vi "q1.vi"() -> ()   [LabVIEW 2015]
panel:
  out "Sin wave":dbl[](graph)=[0.0, 0.06279051952931337, 0.12533323356430426, 0.1873813145857246, 0.2486898871648548, 0.3090169943749474, 0.3681245526846779, 0.4257792915650727, 0.4817536741017153, 0.5358267949789967, 0.5877852522924731, 0.6374239897486896, 0.6845471059286886, 0.7289686274214116, 0.7705132427757893, 0.8090169943749475, 0.8443279255020151, 0.8763066800438637, 0.9048270524660196, 0.9297764858882513, 0.9510565162951535, 0.9685831611286311, 0.9822872507286886, 0.9921147013144779, 0.9980267284282716, 1.0, 0.9980267284282716, 0.9921147013144778, 0.9822872507286886, 0.9685831611286312, 0.9510565162951536, 0.9297764858882515, 0.9048270524660195, 0.8763066800438635, 0.844327925502015, 0.8090169943749475, 0.7705132427757893, 0.7289686274214114, 0.6845471059286888, 0.6374239897486899, 0.5877852522924732, 0.5358267949789967, 0.4817536741017156, 0.4257792915650729, 0.36812455268467814, 0.3090169943749475, 0.24868988716485482, 0.18738131458572457, 0.12533323356430454, 0.06279051952931358, 1.2246467991473532e-16, -0.06279051952931335, -0.12533323356430429, -0.18738131458572477, -0.24868988716485502, -0.30901699437494773, -0.3681245526846783, -0.42577929156507266, -0.481753674101715, -0.5358267949789964, -0.587785252292473, -0.6374239897486896, -0.6845471059286887, -0.7289686274214113, -0.7705132427757894, -0.8090169943749473, -0.8443279255020153, -0.8763066800438636, -0.9048270524660198, -0.9297764858882515, -0.9510565162951535, -0.968583161128631, -0.9822872507286887, -0.9921147013144778, -0.9980267284282716, -1.0, -0.9980267284282716, -0.9921147013144779, -0.9822872507286887, -0.9685831611286311, -0.9510565162951536, -0.9297764858882512, -0.9048270524660196, -0.8763066800438634, -0.8443279255020155, -0.8090169943749476, -0.7705132427757896, -0.7289686274214116, -0.684547105928689, -0.6374239897486896, -0.5877852522924734, -0.5358267949789963, -0.4817536741017153, -0.4257792915650722, -0.36812455268467786, -0.3090169943749477, -0.24868988716485535, -0.18738131458572468, -0.12533323356430465, -0.06279051952931326, -2.4492935982947064e-16, 0.06279051952931278, 0.12533323356430418, 0.1873813145857242, 0.24868988716485488, 0.3090169943749472, 0.3681245526846782, 0.42577929156507255, 0.48175367410171566, 0.5358267949789967, 0.5877852522924736, 0.63742398974869, 0.6845471059286892, 0.7289686274214119, 0.7705132427757893, 0.8090169943749478, 0.8443279255020147, 0.8763066800438631, 0.9048270524660194, 0.9297764858882511, 0.9510565162951535, 0.968583161128631, 0.9822872507286886, 0.9921147013144778, 0.9980267284282716, 1.0, 0.9980267284282716, 0.9921147013144779, 0.9822872507286886, 0.9685831611286311, 0.9510565162951536, 0.9297764858882517, 0.9048270524660192, 0.8763066800438634, 0.8443279255020151, 0.8090169943749476, 0.7705132427757886, 0.728968627421411, 0.6845471059286884, 0.6374239897486897, 0.5877852522924734, 0.5358267949789972, 0.4817536741017162, 0.42577929156507394, 0.368124552684678, 0.3090169943749478, 0.2486898871648555, 0.18738131458572568, 0.1253332335643039, 0.06279051952931339, 3.6739403974420594e-16, -0.06279051952931265, -0.12533323356430318, -0.18738131458572496, -0.24868988716485477, -0.30901699437494706, -0.36812455268467725, -0.42577929156507327, -0.48175367410171555, -0.5358267949789965, -0.5877852522924728, -0.6374239897486905, -0.6845471059286892, -0.7289686274214118, -0.7705132427757891, -0.8090169943749472, -0.8443279255020156, -0.876306680043863, -0.9048270524660189, -0.9297764858882513, -0.9510565162951534, -0.968583161128631, -0.9822872507286885, -0.9921147013144779, -0.9980267284282716, -1.0, -0.9980267284282716, -0.992114701314478, -0.9822872507286886, -0.9685831611286312, -0.9510565162951538, -0.9297764858882517, -0.9048270524660192, -0.8763066800438635, -0.8443279255020152, -0.8090169943749477, -0.7705132427757886, -0.7289686274214111, -0.6845471059286885, -0.6374239897486897, -0.5877852522924735, -0.5358267949789958, -0.4817536741017163, -0.42577929156507405, -0.3681245526846781, -0.3090169943749479, -0.2486898871648556, -0.1873813145857258, -0.125333233564304, -0.06279051952931351, -4.898587196589413e-16, 0.0627905195293143, 0.12533323356430304, 0.18738131458572485, 0.24868988716485466, 0.30901699437494523, 0.36812455268467714, 0.42577929156507155, 0.48175367410171543, 0.535826794978995, 0.5877852522924727, 0.6374239897486891, 0.6845471059286891, 0.7289686274214104, 0.7705132427757891, 0.8090169943749471, 0.8443279255020155, 0.876306680043863, 0.9048270524660196, 0.9297764858882513, 0.951056516295154, 0.9685831611286309, 0.9822872507286888, 0.9921147013144779, 0.9980267284282717, 1.0, 0.9980267284282716, 0.992114701314478, 0.9822872507286886, 0.9685831611286312, 0.9510565162951532, 0.9297764858882518, 0.9048270524660201, 0.8763066800438635, 0.8443279255020162, 0.8090169943749478, 0.7705132427757898, 0.7289686274214111, 0.6845471059286898, 0.6374239897486899, 0.5877852522924736, 0.5358267949789959, 0.48175367410171643, 0.42577929156507255, 0.3681245526846782, 0.3090169943749463, 0.2486898871648557, 0.18738131458572418, 0.12533323356430415, 0.06279051952931186, 6.123233995736766e-16, -0.06279051952931418, -0.12533323356430293, -0.1873813145857247, -0.24868988716485452, -0.3090169943749485, -0.3681245526846787, -0.42577929156506983, -0.4817536741017153, -0.5358267949789963, -0.5877852522924726, -0.637423989748689, -0.6845471059286876, -0.7289686274214103, -0.7705132427757901, -0.809016994374946, -0.8443279255020155, -0.8763066800438638, -0.9048270524660196, -0.9297764858882513, -0.9510565162951534, -0.9685831611286309, -0.982287250728689, -0.9921147013144777, -0.9980267284282717, -1.0, -0.9980267284282716, -0.9921147013144778, -0.9822872507286887, -0.9685831611286312, -0.9510565162951538, -0.9297764858882518, -0.9048270524660201, -0.8763066800438645, -0.8443279255020162, -0.8090169943749468, -0.770513242775791, -0.7289686274214113, -0.6845471059286887, -0.63742398974869, -0.5877852522924737, -0.5358267949789975, -0.48175367410171654, -0.42577929156507105, -0.36812455268468, -0.3090169943749464, -0.2486898871648541, -0.1873813145857243, -0.12533323356430426, -0.06279051952931375, -7.347880794884119e-16, 0.06279051952931583, 0.12533323356430282, 0.18738131458572635, 0.24868988716485269, 0.3090169943749484, 0.3681245526846786, 0.42577929156507294, 0.4817536741017152, 0.5358267949789963, 0.5877852522924725, 0.6374239897486889, 0.6845471059286876, 0.7289686274214102, 0.7705132427757901, 0.8090169943749459, 0.8443279255020154, 0.8763066800438637, 0.9048270524660195, 0.9297764858882512]
  out "Integration Graph":dbl[](graph)=[0.0, 0.00012558103905862674, 0.00037624750618723527, 0.0007510101353586844, 0.001248389909688394, 0.001866423898438289, 0.002602673003807645, 0.0034542315869377904, 0.004417738935141221, 0.005489392525099214, 0.006664963029684161, 0.00793981100918154, 0.009308905221038917, 0.01076684247588174, 0.01230786896143332, 0.013925902950183214, 0.015614558801187244, 0.017367172161274973, 0.019176826266207012, 0.021036379237983516, 0.02293849227057382, 0.024875658592831085, 0.02684023309428846, 0.028824462496917416, 0.03082051595377396, 0.03282051595377396, 0.0348165694106305, 0.036800798813259455, 0.038765373314716835, 0.040702539636974094, 0.042604652669564404, 0.044464205641340904, 0.04627385974627294, 0.04802647310636066, 0.04971512895736469, 0.051333162946114584, 0.05287418943166616, 0.05433212668650898, 0.05570122089836636, 0.056976068877863745, 0.05815163938244869, 0.05922329297240668, 0.060186800320610113, 0.06103835890374026, 0.06177460800910961, 0.06239264199785951, 0.06289002177218922, 0.06326478440136067, 0.06351545086848928, 0.06364103190754791, 0.06364103190754791, 0.06351545086848928, 0.06326478440136067, 0.06289002177218922, 0.06239264199785951, 0.06177460800910961, 0.06103835890374026, 0.060186800320610113, 0.05922329297240669, 0.058151639382448696, 0.05697606887786375, 0.05570122089836637, 0.05433212668650899, 0.05287418943166617, 0.05133316294611459, 0.0497151289573647, 0.04802647310636067, 0.04627385974627295, 0.044464205641340904, 0.042604652669564404, 0.040702539636974094, 0.038765373314716835, 0.036800798813259455, 0.0348165694106305, 0.03282051595377396, 0.030820515953773955, 0.028824462496917412, 0.026840233094288457, 0.024875658592831078, 0.022938492270573815, 0.02103637923798351, 0.019176826266207005, 0.017367172161274966, 0.015614558801187239, 0.013925902950183207, 0.012307868961433311, 0.010766842475881732, 0.009308905221038909, 0.00793981100918153, 0.006664963029684151, 0.005489392525099205, 0.004417738935141212, 0.0034542315869377812, 0.0026026730038076367, 0.001866423898438281, 0.0012483899096883857, 0.000751010135358675, 0.0003762475061872256, 0.0001255810390586163, -1.021860547567588e-17, -1.0708464195334821e-17, 0.00012558103905861484, 0.0003762475061872232, 0.0007510101353586716, 0.0012483899096883814, 0.001866423898438276, 0.0026026730038076324, 0.0034542315869377773, 0.0044177389351412084, 0.005489392525099202, 0.006664963029684149, 0.007939811009181529, 0.009308905221038907, 0.01076684247588173, 0.01230786896143331, 0.013925902950183205, 0.015614558801187235, 0.017367172161274962, 0.019176826266207002, 0.021036379237983505, 0.02293849227057381, 0.024875658592831074, 0.02684023309428845, 0.028824462496917405, 0.03082051595377395, 0.03282051595377395, 0.034816569410630493, 0.03680079881325945, 0.03876537331471683, 0.04070253963697409, 0.0426046526695644, 0.044464205641340904, 0.04627385974627294, 0.04802647310636066, 0.04971512895736469, 0.051333162946114584, 0.05287418943166616, 0.05433212668650898, 0.05570122089836636, 0.056976068877863745, 0.05815163938244869, 0.05922329297240668, 0.060186800320610113, 0.061038358903740264, 0.06177460800910962, 0.062392641997859516, 0.06289002177218923, 0.06326478440136069, 0.0635154508684893, 0.06364103190754793, 0.06364103190754793, 0.0635154508684893, 0.06326478440136069, 0.06289002177218923, 0.06239264199785952, 0.06177460800910963, 0.06103835890374028, 0.060186800320610134, 0.0592232929724067, 0.05815163938244871, 0.056976068877863766, 0.055701220898366384, 0.054332126686509004, 0.05287418943166618, 0.0513331629461146, 0.049715128957364706, 0.04802647310636068, 0.046273859746272954, 0.04446420564134092, 0.04260465266956442, 0.04070253963697411, 0.03876537331471685, 0.03680079881325947, 0.034816569410630514, 0.03282051595377397, 0.03082051595377397, 0.028824462496917426, 0.02684023309428847, 0.024875658592831095, 0.022938492270573832, 0.021036379237983523, 0.01917682626620702, 0.01736717216127498, 0.015614558801187253, 0.013925902950183222, 0.012307868961433327, 0.01076684247588175, 0.009308905221038928, 0.007939811009181551, 0.006664963029684171, 0.005489392525099225, 0.004417738935141233, 0.0034542315869378, 0.002602673003807652, 0.0018664238984382958, 0.0012483899096884, 0.0007510101353586889, 0.00037624750618723727, 0.00012558103905862926, 2.222614453595284e-18, 1.2428970142774016e-18, 0.00012558103905862985, 0.0003762475061872359, 0.0007510101353586856, 0.0012483899096883948, 0.0018664238984382854, 0.0026026730038076398, 0.003454231586937783, 0.004417738935141214, 0.005489392525099204, 0.006664963029684149, 0.007939811009181527, 0.009308905221038905, 0.010766842475881727, 0.012307868961433306, 0.0139259029501832, 0.015614558801187232, 0.01736717216127496, 0.019176826266207, 0.021036379237983502, 0.02293849227057381, 0.024875658592831074, 0.02684023309428845, 0.028824462496917405, 0.03082051595377395, 0.03282051595377395, 0.034816569410630493, 0.03680079881325945, 0.03876537331471683, 0.04070253963697409, 0.0426046526695644, 0.044464205641340904, 0.04627385974627295, 0.04802647310636067, 0.049715128957364706, 0.0513331629461146, 0.05287418943166618, 0.054332126686509, 0.05570122089836638, 0.05697606887786376, 0.0581516393824487, 0.059223292972406694, 0.06018680032061013, 0.06103835890374027, 0.061774608009109624, 0.062392641997859516, 0.06289002177218923, 0.06326478440136069, 0.0635154508684893, 0.06364103190754791, 0.06364103190754791, 0.06351545086848928, 0.06326478440136067, 0.06289002177218922, 0.06239264199785951, 0.06177460800910961, 0.06103835890374025, 0.060186800320610113, 0.05922329297240668, 0.05815163938244869, 0.056976068877863745, 0.05570122089836637, 0.054332126686509, 0.05287418943166618, 0.0513331629461146, 0.049715128957364706, 0.04802647310636068, 0.04627385974627295, 0.04446420564134091, 0.04260465266956441, 0.0407025396369741, 0.03876537331471684, 0.03680079881325946, 0.03481656941063051, 0.032820515953773964, 0.030820515953773962, 0.02882446249691742, 0.026840233094288464, 0.024875658592831085, 0.02293849227057382, 0.021036379237983516, 0.019176826266207012, 0.017367172161274973, 0.015614558801187244, 0.013925902950183212, 0.012307868961433318, 0.010766842475881735, 0.009308905221038912, 0.007939811009181535, 0.006664963029684156, 0.005489392525099208, 0.004417738935141213, 0.00345423158693778, 0.002602673003807638, 0.001866423898438278, 0.0012483899096883853, 0.0007510101353586772, 0.00037624750618722854, 0.00012558103905862004, -7.453889935837843e-18, -8.923466094814667e-18, 0.00012558103905862275, 0.0003762475061872284, 0.0007510101353586811, 0.0012483899096883864, 0.0018664238984382833, 0.0026026730038076406, 0.0034542315869377864, 0.004417738935141217, 0.00548939252509921, 0.006664963029684155, 0.007939811009181532, 0.009308905221038907, 0.010766842475881727, 0.012307868961433308, 0.0139259029501832, 0.01561455880118723, 0.01736717216127496, 0.019176826266207, 0.021036379237983502]
  out "Numeric":dbl=0.021036379237983502
  in  "Amplitude":dbl=1.0
  in  "Fs":dbl=500.0
  in  "phase":dbl
  in  "Frequency":dbl=5.0
  in  "milliseconds to wait":u32
  out "Numeric 3":dbl=319.0
  in  "No of Iteration":i32=320
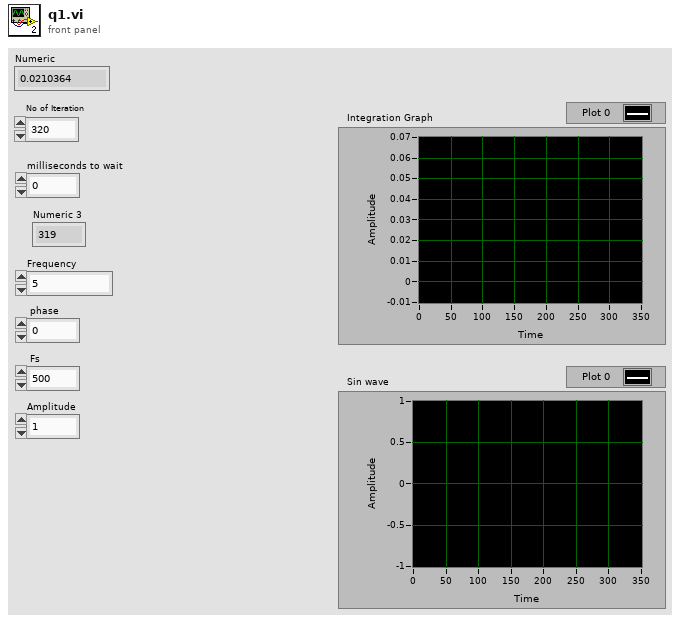
[diagram p1: front panel]
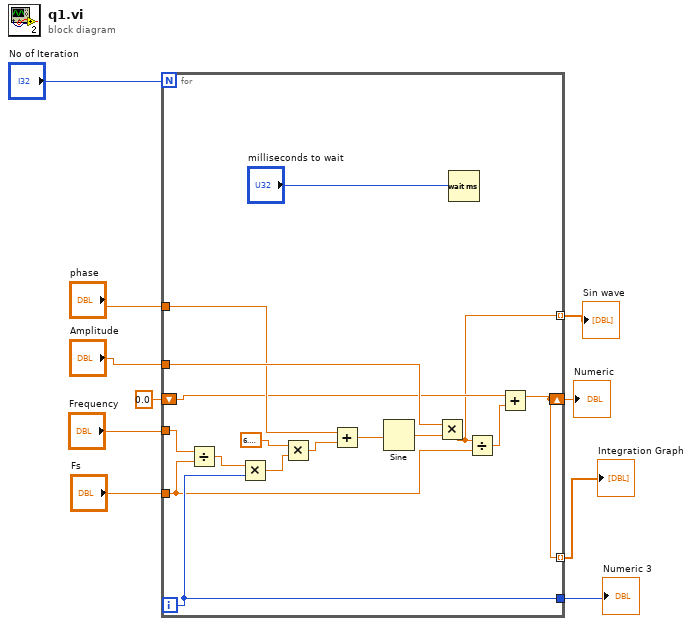
[diagram p0: block diagram]
diagram:
  n1 = for {
    N: "No of Iteration" -> [_]
    tunnel: [w15] -> w10
    tunnel: "Frequency" -> [w24]
    tunnel: "Fs" -> [w13]
    tunnel: "Amplitude" -> [w20]
    tunnel: "phase" -> [w19]
    shift-right: [w11] -> w3
    shift-left: 0.0 -> [w17]
    tunnel: [w11] -> w6 mode=indexing
    tunnel: [w12] -> w2 mode=indexing
    i -> [w15]
    n2 = Divide(x=w24, y=w13) -> (x/y=w18:dbl)
    n3 = Multiply(x=w18, y=w15) -> (x*y=w22:dbl)
    n4 = Multiply(x=6.283185307179586, y=w22) -> (x*y=w23:dbl)
    n5 = Add(x=w19, y=w23) -> (x+y=w25:dbl)
    n6 = Sine(x=w25) -> (sin(x)=w21:dbl)
    n7 = Multiply(x=w20, y=w21) -> (x*y=w12:dbl)
    n8 = Wait (ms)(milliseconds to wait="milliseconds to wait") -> ()  [unwired: 1 out]
    n9 = Divide(x=w12, y=w13) -> (x/y=w14:dbl)
    n10 = Add(x=w17, y=w14) -> (x+y=w11:dbl)
  }
  "Numeric 3" <- w10
  "Numeric" <- w3
  "Integration Graph" <- w6
  "Sin wave" <- w2
